vi "BasicControlCall.vi"(2 "Code":string="x=plantState[1];\ncontrolState[0]=-x;\nfor (i=0; i<200000000 ; i++);", 3 "plantState":dbl[](array[numeric])=[1.0, 6.74]) -> (0 "error":errorcluster={"status"=TRUE, "code"=-2147467259, "source"="Exception occured in ScriptControl: The script was aborted because execution exceeded the specified timeout period.Help Path is MSSCRIPT.HLP and context 0 in BasicControlCall.vi->Test.vi"}, 1 "controlState":dbl[](array[numeric]))   [LabVIEW 2013]
panel:
  in  "Timeout":i32=500
  out "LastCode":string="x=plantState[1];\ncontrolState[0]=-x;\nfor (i=0; i<200000000 ; i++);"
  out "textControlState":string
  out "FullCode":string="function Conversions(textPlantState,textControlState)\n{\nvar plantState=textPlantState.split(\",\");\nfor(var i = 0; i < plantState.length; ++i)\n{plantState[i]=Number(plantState[i]);}  \nvar controlState=textControlState.split(\",\");\nfor(i = 0; i < controlState.length; ++i)\n{controlState[i]=Number(controlState[i]);}\ncontolState=Controller(plantState,controlState);\nreturn contolState.toString();\n}\n\nfunction Controller(plantState,controlState)\n{\nx=plantState[1];\ncontrolState[0]=-x;\nfor (i=0; i<200000000 ; i++);\nreturn controlState;\n}"
  out "textPlantState":string="1.000000E+0,6.740000E+0"
  in  "ScriptControl":refnum<k7>(container)
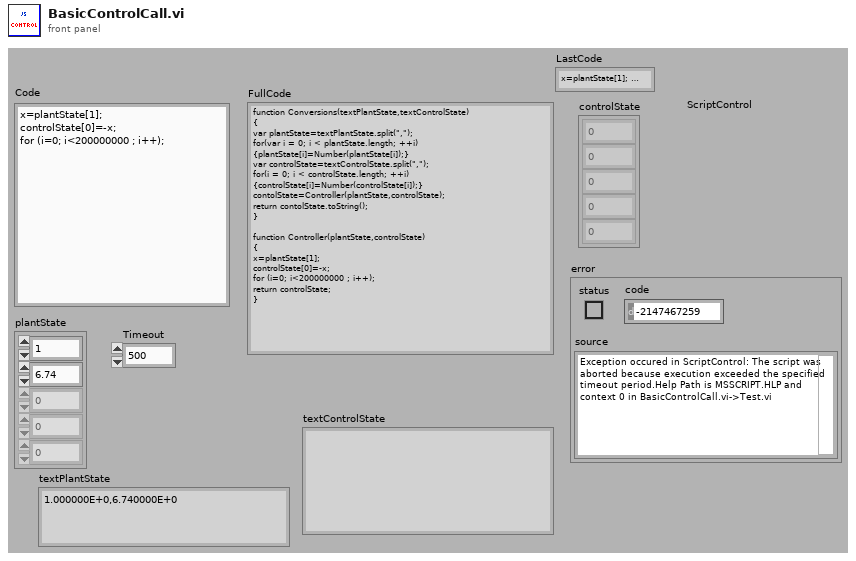
[diagram p1: front panel]
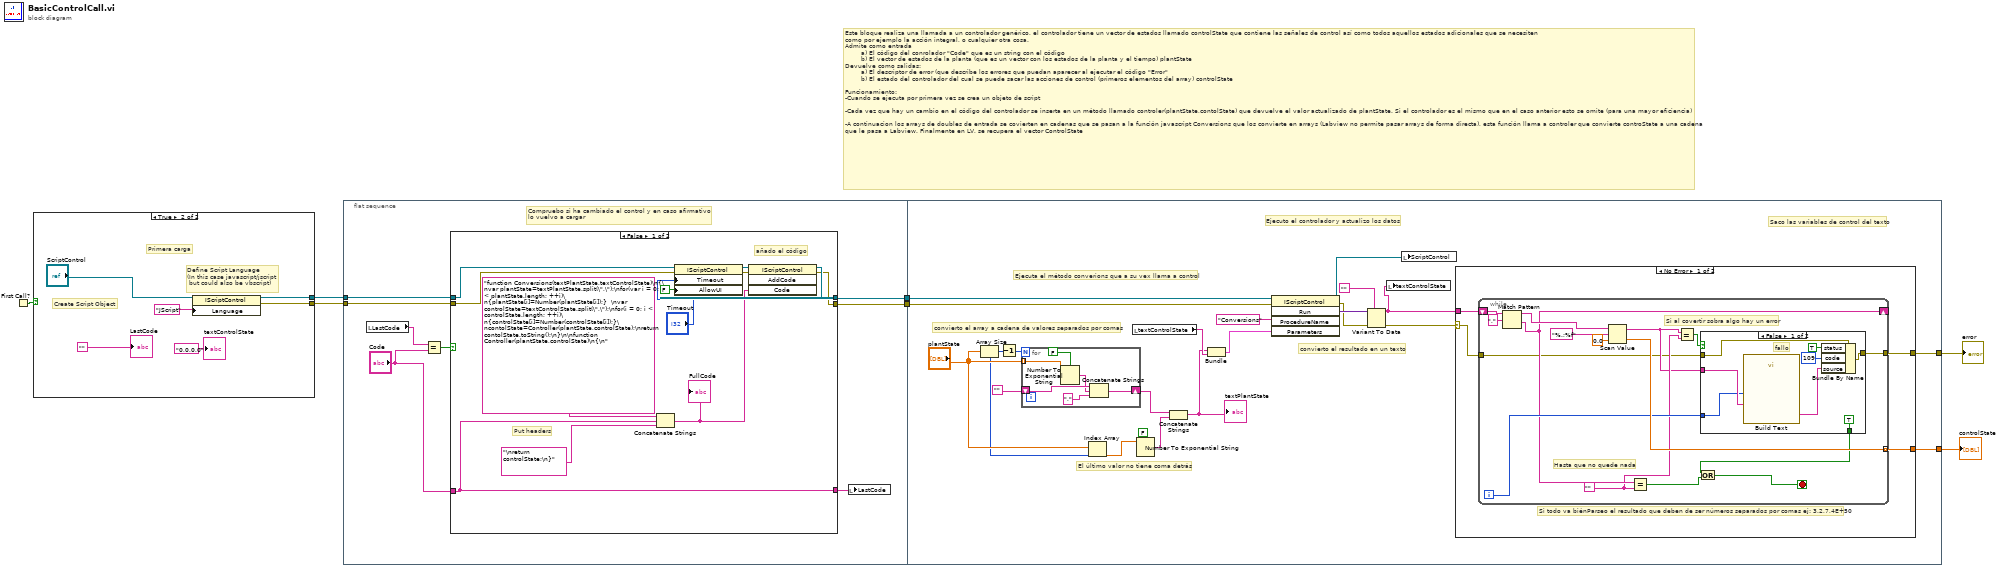
[diagram p0: block diagram]
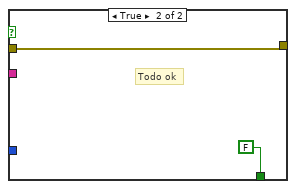
[diagram p3: hidden frame]
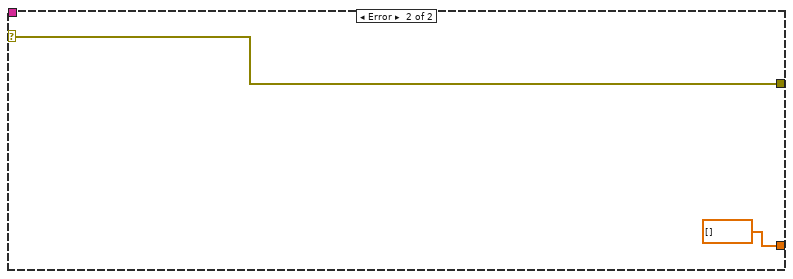
[diagram p4: hidden frame]
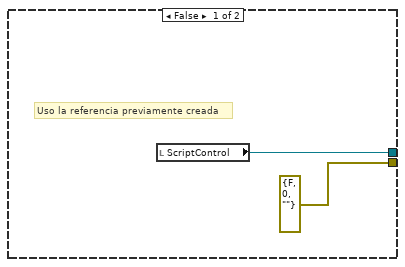
[diagram p5: hidden frame]
diagram:
  # "Este bloque realiza una llamada a un controlador genérico, el controlador tiene un vector de estados llamado controlState que contiene las señales de control así como todos aquellos estados adicionales que se necesiten\ncomo por ejemplo la acción integral, o cualquier otra cosa.\nAdmite como entrada \n        a) El código del conrolador \"Code\" que es un string con el código \n        b) El vector de estados de la planta (que es un vector con los estados de la planta y el tiempo) plantState\nDevuelve como salidas:\n        a) El descriptor de error (que describe los errores que puedan aparecer al ejecutar el código \"Error\"\n        b) El estado del controlador del cual se puede sacar las acciones de control (primeros elementos del array) controlState\n\nFuncionamiento:\n-Cuando se ejecuta por primera vez se crea un objeto de script\n\n-Cada vez que hay un cambio en el código del controlador se inserta en un método llamado controler(plantState,contolState) que devuelve el valor actualizado de plantState. Si el controlador es el mismo que en el caso anterior esto se omite (para una mayor eficiencia)\n \n-A continuacion los arrays de doubles de entrada se covierten en cadenas que se pasan a la función javascript Conversions que los convierte en arrays (Labview no permite pasar arrays de forma directa), esta función llama a controler que convierte controState a una cadena\nque le pasa a Labview. Finalmente en LV, se recupera el vector ControlState"
  n1 = First Call?() -> (First Call?: T/F=w7:bool)
  n2 = case shown="True" w7 {
    tunnel: [w9 w12] -> w6
    tunnel: [errorcluster {"status"=FALSE, "code"=0, "source"=""} ("error out") w11] -> w2
    frame False {
      # "Uso la referencia previamente creada"
      n3 = local read "ScriptControl"() -> (w9:refnum<k7>)
    }
    frame True {
      # "Create Script Object"
      # "Define Script Language\n(In this case javascript/jscript\n but could also be vbscript)"
      # "Primera carga"
      n4 = property class="IScriptControl"(reference="ScriptControl", "Language"="JScript") -> (reference out=w12:refnum<k7>, error out=w11:errorcluster)  [unwired: 1 in]
      "LastCode" <- ""
      "textControlState" <- "0,0,0,0" ("textControlState")
    }
  }
  n5 = flat-sequence {
    tunnel: w6 -> [w20]
    tunnel: [w21] -> w5
    tunnel: w2 -> [w17]
    tunnel: [w16] -> w1
    tunnel: w5 -> [w41]
    tunnel: [w44] -> w4
    tunnel: [w43] -> w3
    tunnel: w1 -> [w40]
    frame #0 {
      # "Compruebo si ha cambiado el control y en caso afirmativo\nlo vuelvo a cargar"
      n6 = local read "LastCode"() -> (w23:string)
      n7 = Equal?(x=w23, y="Code") -> (x = y?=w22:bool)
      n8 = case shown="False" w22 {
        tunnel: [w32 w38] -> w21
        tunnel: w20 -> [w27 w38]
        tunnel: "Code" -> [w31 w37]
        tunnel: [w31 w37] -> w18
        tunnel: w17 -> [w26 w36]
        tunnel: [w30 w36] -> w16
        frame False {
          # "Put headers"
          # "añado el código"
          n9 = Concatenate Strings("function Conversions(textPlantState,textControlState)\n{\nvar plantState=textPlantState.split(\",\");\nfor(var i = 0; i < plantState.length; ++i)\n{plantState[i]=Number(plantState[i]);}  \nvar controlState=textControlState.split(\",\");\nfor(i = 0; i < controlState.length; ++i)\n{controlState[i]=Number(controlState[i]);}\ncontolState=Controller(plantState,controlState);\nreturn contolState.toString();\n}\n\nfunction Controller(plantState,controlState)\n{\n" ("string"), w31, "\nreturn controlState;\n}" ("string")) -> (w35:string)
          "FullCode" <- w35
          n10 = property class="IScriptControl"(reference=w27, error in=w26, "Timeout"="Timeout", "AllowUI"=FALSE) -> (reference out=w28:refnum<k7>, error out=w25:errorcluster)
          n11 = invoke class="IScriptControl" method="AddCode"(reference=w28, error in=w25, "Code"=w35) -> (reference out=w32:refnum<k7>, error out=w30:errorcluster)  [unwired: 1 in, 2 out]
        }
        frame True {
          # "No hago nada"
        }
      }
      n12 = local write "LastCode"(w18) -> ()
    }
    frame #1 {
      # "Saco las variables de control del texto"
      # "convierto el resultado en un texto"
      # "El último valor no tiene coma detrás"
      # "convierto el array a cadena de valores separados por comas"
      # "Ejecuta el método converions que a su vex llama a control"
      # "Ejecuto el controlador y actualizo los datos"
      n13 = Array Size(array="plantState") -> (size(s)=w54:i32)
      n14 = Decrement(x=w54) -> (x-1=w55:i32)
      n15 = for {
        N: w55 -> [_]
        tunnel: "plantState" -> [w98] mode=indexing
        shift-right: [w96] -> w49
        shift-left: "" -> [w94]
        n16 = Number To Exponential String(number=w98, 1:FALSE ("use system decimal point (T)")) -> (E-format string=w93:string)  [unwired: 2 in]
        n17 = Concatenate Strings(w94, w93, "," ("string")) -> (w96:string)
      }
      n18 = Index Array(array="plantState", index=w55) -> (element=w52:dbl)
      n19 = local read "textControlState"() -> (w50:string)
      n20 = Number To Exponential String(number=w52, 1:FALSE ("use system decimal point (T)")) -> (E-format string=w53:string)  [unwired: 2 in]
      n21 = Concatenate Strings(w49, w53) -> (w48:string)
      "textPlantState" <- w48
      n22 = Bundle(w48, "textControlState"=w50) -> (w58:cluster{string, "textControlState":string})  [unwired: 1 in]
      n23 = invoke class="IScriptControl" method="Run"(reference=w41, error in=w40, "ProcedureName"="Conversions", "Parameters"=w58) -> (reference out=w39:refnum<k7>, error out=w45:errorcluster, "Run"=w46:variant)  [unwired: 1 in, 2 out]
      n24 = Variant To Data(error in=w45, type="", Variant=w46) -> (data=w42:string, error out=w60:errorcluster)
      n25 = local write "textControlState"(w42) -> ()
      n26 = local write "ScriptControl"(w39) -> ()
      n27 = case shown="No Error" w60 {
        selector: w60 -> [w61 w92]
        tunnel: [w64 dbl[] [] ("Array")] -> w43
        tunnel: w42 -> [w63 _]
        tunnel: [w62 w92] -> w44
        frame No Error {
          # "Si todo va biénParseo el resultado que deben de ser números separados por comas ej: 3.2,7,4E+50"
          n28 = while {
            shift-right: [w69] -> _
            shift-left: w63 -> [w79]
            tunnel: [w77] -> w64 mode=indexing
            tunnel: [w71] -> w62
            tunnel: w61 -> [w65]
            i -> [w74]
            stop <- w72 stop-if-true
            w68 = ""
            # "Hasta que no quede nada"
            # "Si al covertir sobra algo hay un error"
            n29 = Match Pattern(string=w79, regular expression=",") -> (before substring=w70:string, after substring=w69:string)  [unwired: 1 in, 2 out]
            n30 = Scan Value(string=w70, format string="%.;%f", default (0 dbl)=0.0) -> (output string=w67:string, value=w77:dbl)
            n31 = Equal?(x=w69, y=w68) -> (x = y?=w73:bool)
            n32 = Equal?(x=w67, y=w68) -> (x = y?=w66:bool)
            n33 = case shown="False" w66 {
              tunnel: [TRUE ("x = y?") FALSE ("x = y?")] -> w75
              tunnel: w74 -> [w82 _]
              tunnel: w67 -> [w88 _]
              tunnel: [w86 w89] -> w71
              tunnel: w65 -> [w81 w89]
              frame False {
                # "fallo"
                n34 = call "Build Text"("num"=w82, "texto"=w88) -> ("Result"=w85:string)  [unwired: 12 in, 1 out]
                n35 = Bundle By Name(cluster=w81, "status"=TRUE, "code"=109, "source"=w85) -> (w86:errorcluster)
              }
              frame True {
                # "Todo ok"
              }
            }
            n36 = Or(x=w75, y=w73) -> (x .or. y?=w72:bool)
          }
        }
        frame Error {
        }
      }
    }
  }
  "error" <- w4
  "controlState" <- w3
